vi "LVCAM Destroy.vi"(10 "Error":errorcluster, 11 "Process in":refnum<class "ABD.lvclass">) -> ()   [LabVIEW 2021, in "ABD.lvlib" / "ABD.lvclass"]
uses:
  ABD.lvclass
  ABD.lvclass/ABD.ctl
  LVCAM/LVCAM/LVCAM/LVCAM.lvclass
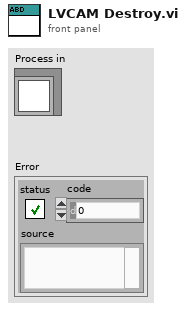
[diagram p1: front panel]
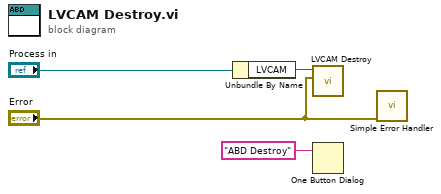
[diagram p0: block diagram]
diagram:
  n1 = Unbundle By Name("Process in") -> ("LVCAM"=w4:refnum<class "LVCAM.lvclass">)
  n2 = call-dynamic "LVCAM Destroy.vi"("Error"="Error", "LVCAM Destroy in"=w4) -> ()  [unwired: 10 in]
  n3 = One Button Dialog(message="ABD Destroy") -> ()  [unwired: 1 in, 1 out]
  n4 = call <vilib>:"Simple Error Handler.vi"("error in (no error)"="Error") -> ()  [unwired: 4 in, 5 out]
